vi "Set Measurement Type.vi"(8 "error in (no error)":errorcluster, 10 "Measurement Type":T1=10 items=["Continuity", "Current AC", "Current DC", "Diode", "Frequency", "Resistance 4-wire", "Period", "Resistance 2-wire", "Temperature", "Voltage AC", "Voltage DC", "Voltage DC Ratio", "Capacitance"], 11 "3446X in":refnum<class "3446X.lvclass">) -> (0 "error out":errorcluster, 3 "3446X out":refnum<class "3446X.lvclass">)   [LabVIEW 2018, in "3446X.lvlib" / "3446X.lvclass"]
doc: "This Overriden is meant to be used/called from the 'Set Measurement Properties.vi' Method, as it ensures several additional properties are properly configured."
uses:
  3446X.lvclass
  PPLs/DMM/Parent/DMM.lvlibp/Custom Controls/Measurement Type.ctl
  3446X.lvclass/3446X.ctl
  <instrlib>/Agilent 3446X Series/Agilent 3446X Series.lvlib
  PPLs/DMM/Parent/DMM.lvlibp/DMM.lvclass
  C:/Projects/LabVIEW/PPLs/DMM/Parent/DMM.lvlibp/DMM.lvclass
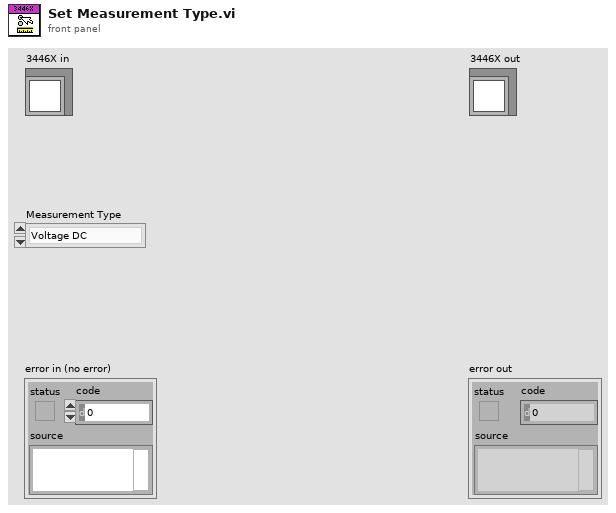
[diagram p1: front panel]
types:
  T1 = typedef "DMM.lvlibp/DMM.lvclass/Measurement Type.ctl" = u32
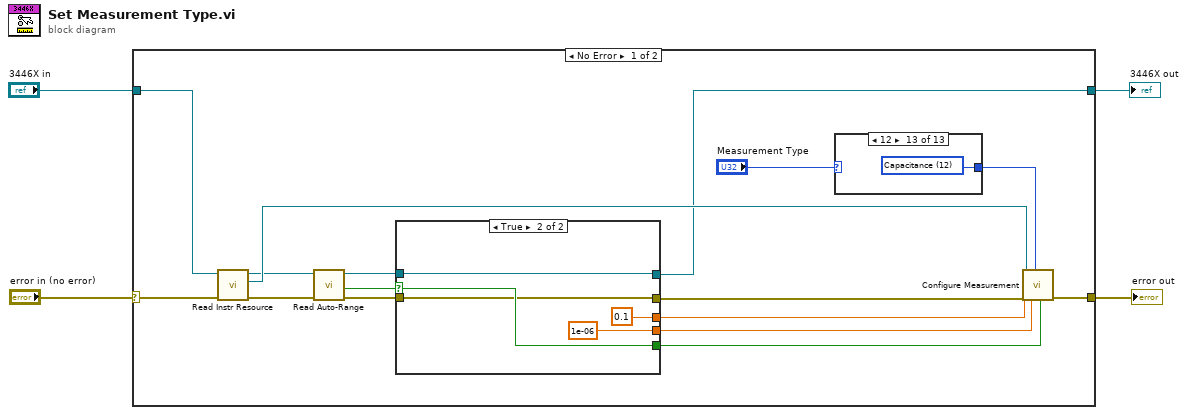
[diagram p0: block diagram]
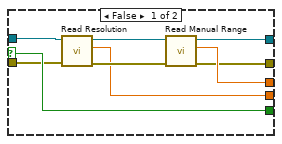
[diagram p2: hidden frame]
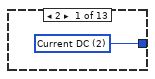
[diagram p3: hidden frame]
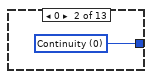
[diagram p4: hidden frame]
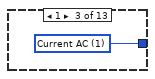
[diagram p5: hidden frame]
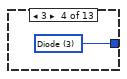
[diagram p6: hidden frame]
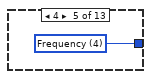
[diagram p7: hidden frame]
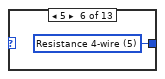
[diagram p8: hidden frame]
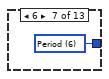
[diagram p9: hidden frame]
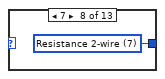
[diagram p10: hidden frame]
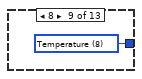
[diagram p11: hidden frame]
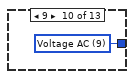
[diagram p12: hidden frame]
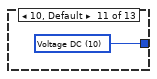
[diagram p13: hidden frame]
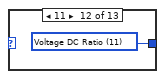
[diagram p14: hidden frame]
diagram:
  n1 = case shown="No Error" "error in (no error)" {
    selector: "error in (no error)" -> [w20 w48]
    tunnel: [w7 w49] -> w3
    tunnel: "3446X in" -> [w19 w49]
    tunnel: [w16 w48] -> w2
    frame No Error {
      n2 = call "Read Instr Resource.vi"("error in (no error)"=w20, "3446X in"=w19) -> ("error out"=w13:errorcluster, "Instr Resource"=w17:refnum<visa-resource-name>, "3446X out"=w14:refnum<class "3446X.lvclass">)  [unwired: 7 in]
      n3 = call "Read Auto-Range.vi"("error in (no error)"=w13, "DMM in"=w14) -> ("error out"=w10:errorcluster, "Auto-Range"=w12:bool, "DMM out"=w8:refnum<class "3446X.lvclass">)  [unwired: 7 in]
      n4 = case shown="True" w12 {
        selector: w12 -> [w29 w34]
        tunnel: [w29 w34] -> w11
        tunnel: w10 -> [w21 w33]
        tunnel: [w27 w33] -> w9
        tunnel: w8 -> [w23 w30]
        tunnel: [w26 w30] -> w7
        tunnel: [w28 0.1 ("Manual Range")] -> w6
        tunnel: [w24 1e-06 ("Absolute Resolution (1E-6)")] -> w5
        frame False {
          n5 = call "Read Resolution.vi"("error in (no error)"=w21, "DMM in"=w23) -> ("error out"=w25:errorcluster, "Resolution"=w24:dbl, "DMM out"=w22:refnum<class "3446X.lvclass">)  [unwired: 7 in]
          n6 = call "Read Manual Range.vi"("error in (no error)"=w25, "DMM in"=w22) -> ("error out"=w27:errorcluster, "Manual Range"=w28:dbl, "DMM out"=w26:refnum<class "3446X.lvclass">)  [unwired: 7 in]
        }
        frame True {
        }
      }
      n7 = case shown="12" "Measurement Type" {
        tunnel: [w35 w36 w37 w38 w39 w40 w41 w42 w43 w44 w45 w46 w47] -> w18
        frame 2 {
          w35 = 2 items=["Continuity", "Current AC", "Current DC", "Diode", "Frequency", "Resistance 4-wire", "Period", "Resistance 2-wire", "Temperature", "Voltage AC", "Voltage DC", "Voltage DC Ratio", "Capacitance"] ("Measurement Function (10: Voltage DC)")
        }
        frame 0 {
          w36 = 0 items=["Continuity", "Current AC", "Current DC", "Diode", "Frequency", "Resistance 4-wire", "Period", "Resistance 2-wire", "Temperature", "Voltage AC", "Voltage DC", "Voltage DC Ratio", "Capacitance"] ("Measurement Function (10: Voltage DC)")
        }
        frame 1 {
          w37 = 1 items=["Continuity", "Current AC", "Current DC", "Diode", "Frequency", "Resistance 4-wire", "Period", "Resistance 2-wire", "Temperature", "Voltage AC", "Voltage DC", "Voltage DC Ratio", "Capacitance"] ("Measurement Function (10: Voltage DC)")
        }
        frame 3 {
          w38 = 3 items=["Continuity", "Current AC", "Current DC", "Diode", "Frequency", "Resistance 4-wire", "Period", "Resistance 2-wire", "Temperature", "Voltage AC", "Voltage DC", "Voltage DC Ratio", "Capacitance"] ("Measurement Function (10: Voltage DC)")
        }
        frame 4 {
          w39 = 4 items=["Continuity", "Current AC", "Current DC", "Diode", "Frequency", "Resistance 4-wire", "Period", "Resistance 2-wire", "Temperature", "Voltage AC", "Voltage DC", "Voltage DC Ratio", "Capacitance"] ("Measurement Function (10: Voltage DC)")
        }
        frame 5 {
          w40 = 5 items=["Continuity", "Current AC", "Current DC", "Diode", "Frequency", "Resistance 4-wire", "Period", "Resistance 2-wire", "Temperature", "Voltage AC", "Voltage DC", "Voltage DC Ratio", "Capacitance"] ("Measurement Function (10: Voltage DC)")
        }
        frame 6 {
          w41 = 6 items=["Continuity", "Current AC", "Current DC", "Diode", "Frequency", "Resistance 4-wire", "Period", "Resistance 2-wire", "Temperature", "Voltage AC", "Voltage DC", "Voltage DC Ratio", "Capacitance"] ("Measurement Function (10: Voltage DC)")
        }
        frame 7 {
          w42 = 7 items=["Continuity", "Current AC", "Current DC", "Diode", "Frequency", "Resistance 4-wire", "Period", "Resistance 2-wire", "Temperature", "Voltage AC", "Voltage DC", "Voltage DC Ratio", "Capacitance"] ("Measurement Function (10: Voltage DC)")
        }
        frame 8 {
          w43 = 8 items=["Continuity", "Current AC", "Current DC", "Diode", "Frequency", "Resistance 4-wire", "Period", "Resistance 2-wire", "Temperature", "Voltage AC", "Voltage DC", "Voltage DC Ratio", "Capacitance"] ("Measurement Function (10: Voltage DC)")
        }
        frame 9 {
          w44 = 9 items=["Continuity", "Current AC", "Current DC", "Diode", "Frequency", "Resistance 4-wire", "Period", "Resistance 2-wire", "Temperature", "Voltage AC", "Voltage DC", "Voltage DC Ratio", "Capacitance"] ("Measurement Function (10: Voltage DC)")
        }
        frame 10, Default {
          w45 = 10 items=["Continuity", "Current AC", "Current DC", "Diode", "Frequency", "Resistance 4-wire", "Period", "Resistance 2-wire", "Temperature", "Voltage AC", "Voltage DC", "Voltage DC Ratio", "Capacitance"] ("Measurement Function (10: Voltage DC)")
        }
        frame 11 {
          w46 = 11 items=["Continuity", "Current AC", "Current DC", "Diode", "Frequency", "Resistance 4-wire", "Period", "Resistance 2-wire", "Temperature", "Voltage AC", "Voltage DC", "Voltage DC Ratio", "Capacitance"] ("Measurement Function (10: Voltage DC)")
        }
        frame 12 {
          w47 = 12 items=["Continuity", "Current AC", "Current DC", "Diode", "Frequency", "Resistance 4-wire", "Period", "Resistance 2-wire", "Temperature", "Voltage AC", "Voltage DC", "Voltage DC Ratio", "Capacitance"] ("Measurement Function (10: Voltage DC)")
        }
      }
      n8 = call <instrlib>:"Configure Measurement.vi"("Manual Range (1)"=w6, "Absolute Resolution (1E-6)"=w5, "error in (no error)"=w9, "Auto Range (T: Enable)"=w11, "Measurement Function (10: Voltage DC)"=w18, "VISA resource name"=w17) -> ("error out"=w16:errorcluster)  [unwired: 4 in, 1 out]
    }
    frame Error {
    }
  }
  "error out" <- w2
  "3446X out" <- w3
